vi "Read cell.vi"(8 "error in (no error)":errorcluster, 11 "Filter Step in":refnum<class "Filter Step.lvclass">) -> (0 "error out":errorcluster, 2 "cell":u8, 3 "Filter Step out":refnum<class "Filter Step.lvclass">)   [LabVIEW 2017, in "Controller.lvlib" / "Filter Step.lvclass"]
uses:
  Filter Step.lvclass
  Filter Step.lvclass/Filter Step.ctl
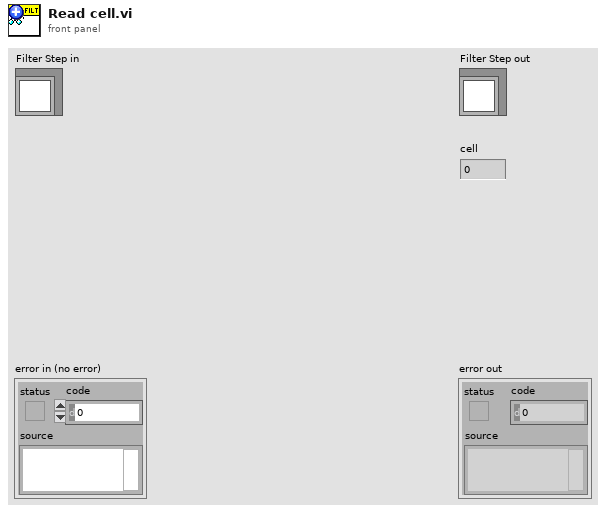
[diagram p1: front panel]
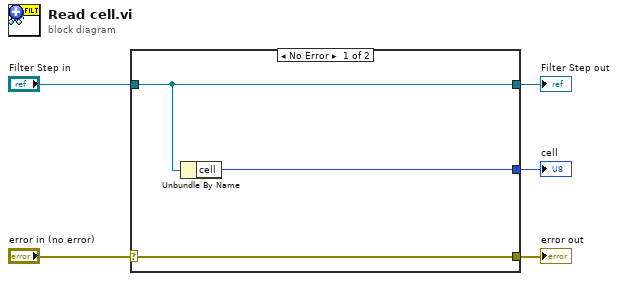
[diagram p0: block diagram]
diagram:
  n1 = case shown="No Error" "error in (no error)" {
    selector: "error in (no error)" -> [w8 w9]
    tunnel: [w8 w9] -> w4
    tunnel: [w7 w10] -> w2
    tunnel: "Filter Step in" -> [w7 w10]
    tunnel: [w6 _] -> w1
    frame No Error {
      n2 = Unbundle By Name(w7) -> ("cell"=w6:u8)
    }
    frame Error {
    }
  }
  "error out" <- w4
  "Filter Step out" <- w2
  "cell" <- w1
